vi "Check Green and Red LED.vi"(6 "error in":errorcluster, 8 "R4012":dbl=2000.0, 9 "R4006":dbl=750.0, 10 "R4001":dbl=1500.0, 11 "DMM":refnum<visa-resource-name>="COM1") -> (0 "error out":errorcluster, 1 "Currents":dbl[](array[numeric]))   [LabVIEW 2015]
uses:
  <instrlib>/Keithley 27XX/Keithley 27XX.lvlib
panel:
  out "Measurement Data":dbl[](array[numeric])
  out "D4 Red Current (mA)":dbl format="%#.2f"
  out "D4 Red OFF":bool
  out "Current (mA) R2012":dbl format="%#.2g"
  out "D4 Red On":bool
  out "Current (mA) R2001":dbl format="%#.2g"
  out "Voltage T7":dbl format="%0.2f"
  out "D4 Green Off":bool
  out "D4 Green On":bool
  in  "Min Led Current":dbl=0.001
  out "D4 Green Current (mA)":dbl format="%#.2f"
  out "Voltage T5":dbl format="%0.2f"
  out "Voltage T6":dbl format="%0.2f"
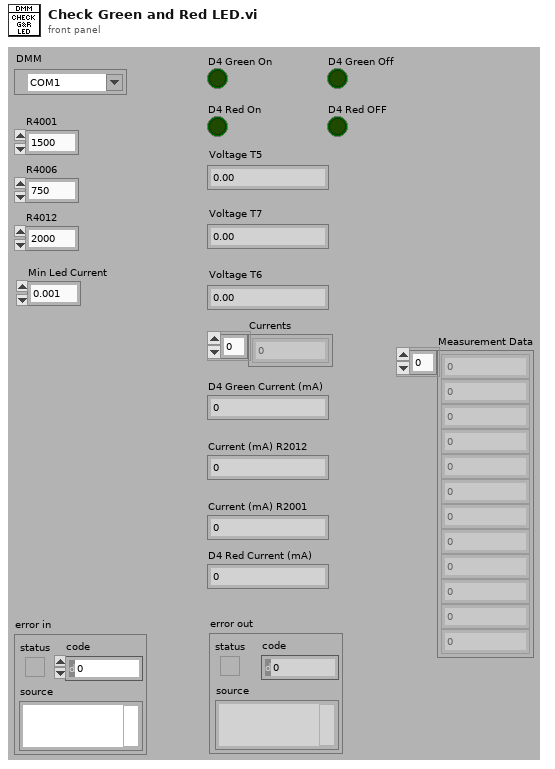
[diagram p1: front panel]
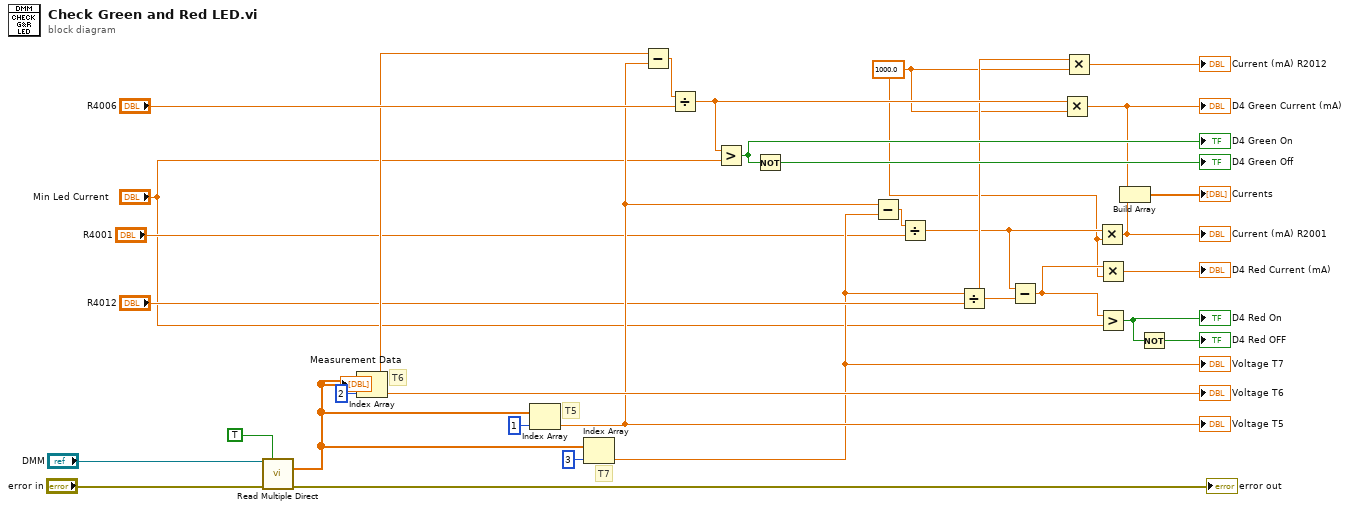
[diagram p0: block diagram]
diagram:
  w10 = 1000.0 ("y")
  # "T7"
  # "T5"
  # "T6"
  n1 = call <instrlib>:"Read Multiple Direct.vi"("VISA resource name"="DMM", "All Data Elements (False)"=TRUE, "error in (no error)"="error in") -> ("Measurement Data"=w4:dbl[], "error out"=→"error out":errorcluster)  [unwired: 7 in, 4 out]
  "Measurement Data" <- w4
  n2 = Index Array(array=w4, index=2) -> (element=w24:dbl)
  "Voltage T6" <- w24
  n3 = Index Array(array=w4, index=1) -> (element=w19:dbl)
  "Voltage T5" <- w19
  n4 = Index Array(array=w4, index=3) -> (element=w17:dbl)
  "Voltage T7" <- w17
  n5 = Subtract(x=w24, y=w19) -> (x-y=w31:dbl)
  n6 = Divide(x=w31, y="R4006") -> (x/y=w27:dbl)
  n7 = Greater?(x=w27, y="Min Led Current") -> (0:w29:bool)
  "D4 Green On" <- w29
  n8 = Not(x=w29) -> (.not. x?=→"D4 Green Off":bool)
  n9 = Subtract(x=w19, y=w17) -> (x-y=w22:dbl)
  n10 = Divide(x=w22, y="R4001") -> (x/y=w12:dbl)
  n11 = Divide(x=w17, y="R4012") -> (x/y=w16:dbl)
  n12 = Subtract(x=w12, y=w16) -> (x-y=w11:dbl)
  n13 = Multiply(x=w27, y=w10) -> (x*y=w8:dbl)
  "D4 Green Current (mA)" <- w8
  n14 = Multiply(x=w16, y=w10) -> (x*y=→"Current (mA) R2012":dbl)
  n15 = Multiply(x=w12, y=w10) -> (x*y=w7:dbl)
  "Current (mA) R2001" <- w7
  n16 = Multiply(x=w11, y=w10) -> (x*y=→"D4 Red Current (mA)":dbl)
  n17 = Greater?(x=w11, y="Min Led Current") -> (0:w21:bool)
  "D4 Red On" <- w21
  n18 = Build Array(w8, w7) -> (→"Currents":dbl[])
  n19 = Not(x=w21) -> (.not. x?=→"D4 Red OFF":bool)
